vi "Background_MC_Acquire_v2.vi"(7 "prev deleted portion":u16[](array[numeric]), 8 "error in":errorcluster, 9 "Image In":T2, 10 "Frames":i16, 11 "FPGA VI Reference In":T1) -> (0 "error out":errorcluster, 1 "deleted portion":u16[](array[numeric]), 2 "Image":T2(plugin-control), 3 "FPGA VI Reference Out":T1)   [LabVIEW 2020]
uses:
  RIG-SPECIFIC FILES/FPGA Refs/FPGA Ref.ctl
  <vilib>/vision/Image Controls.llb/IMAQ Image.ctl
  <vilib>/Utility/error.llb/Error Cluster From Error Code.vi
  <vilib>/rvi/errors/niLvFpgaAdjustHostInterfaceError.vi
  <vilib>/rvi/interface/nirviMethod/nirviMethod.xnode
  <vilib>/FPGAPlugInAG/Dynamic/niLvFpga_ReadFifo_Dynamic.vi
  <vilib>/rvi/errors/niLvFpgaMergeErrorWithErrorCode.vi
panel:
  out "deleted ele":i32
  out "1D Array incoming":i32
  out "1D Array size Adj":i32(graph)
  out "1D Array incoming":cluster{"Total number of pixels":i16, i32}(graph)
  out "Final Array size":i32[](array[numeric])
  out "Reshaped Array size":i32[](array[numeric])
  out "1D Array size":i32
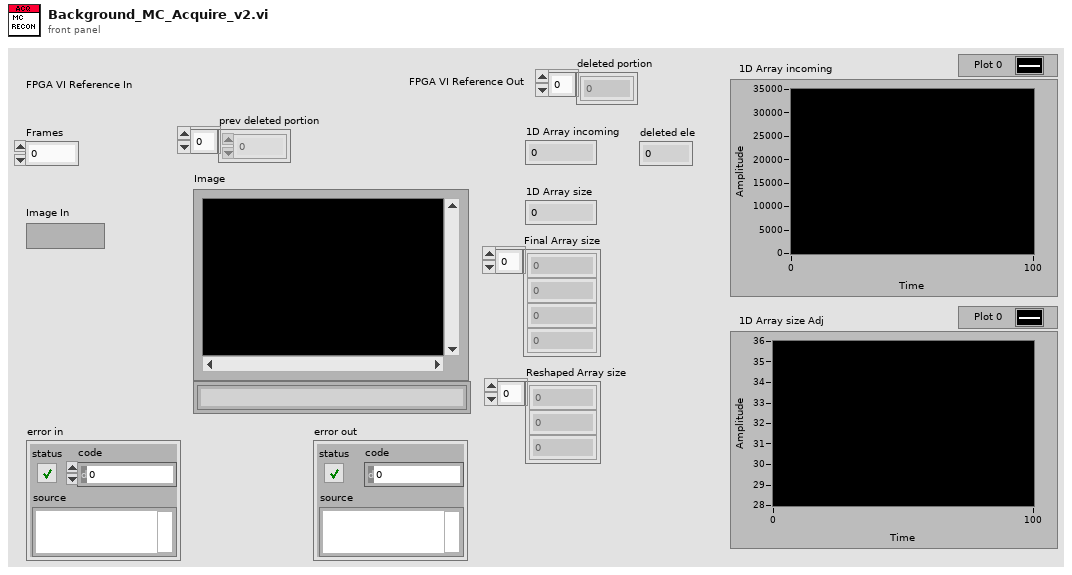
[diagram p1: front panel]
types:
  T1 = typedef "FPGA Ref.ctl" = refnum<k20>
  T2 = typedef "IMAQ Image.ctl" = refnum<image>
  T3 = typedef "Ref DAQ Param.ctl" = cluster{"Full Frame Size":u16, "Ref Field of View":sgl, "Ref Zoom":i8, "Ref_dwellTime":sgl, "Ref X-pixels-per-line(Npxr)":i16, "Ref Y-lines-per-image(Npyr)":i16, "Ref Z-lines-per-image":i16, "Ignore Z lines":i16, "Ref Scan Cycles":i32, "Ref threshold XY":u16, "Ref threshold Z":u16, "Ref average XY":u16, "Ref Average  Z":u16, "Proportional_scale":fxp<+,16,2>, "Integral_scale":fxp<+/-,16,12>, "Proportional_scale Z":fxp<+,16,2>, "Integral_scale Z":fxp<+/-,16,12>, "Diff_threshold":fxp<+,16,2>, "Diff_threshold _z":fxp<+,16,2>, "Sliding Average":bool, "Ref count reset enabled":bool, "Auto-centering":bool}
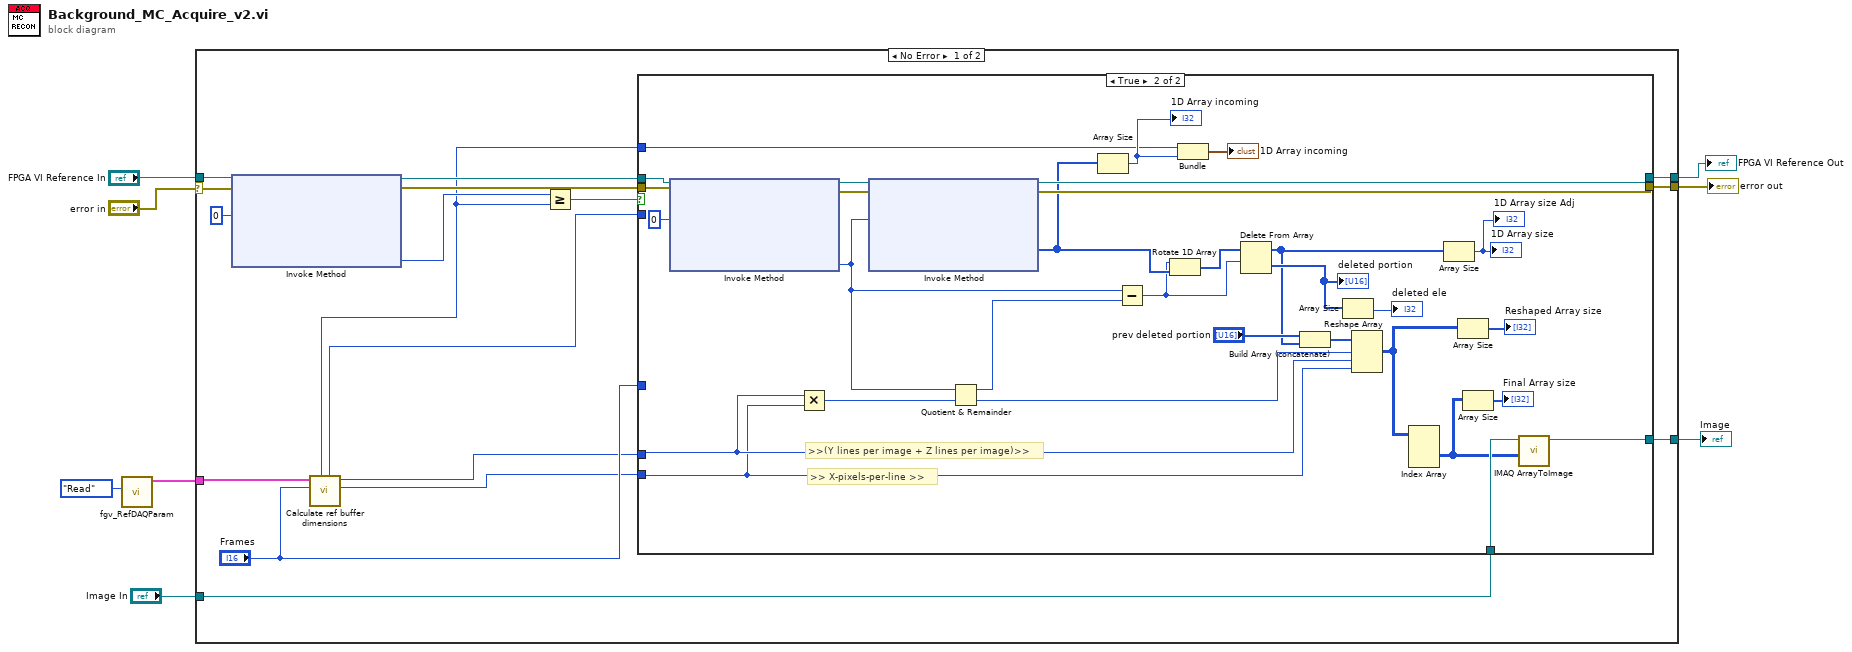
[diagram p0: block diagram]
diagram:
  n1 = call "fgv_RefDAQParam.vi"("Function"=enum16{"Initialize", "Write", "Read"}."Read") -> ("RefDAQParam"=w5:T3)  [unwired: 9 in, 1 out]
  n2 = case shown="No Error" "error in" {
    selector: "error in" -> [w23 w59]
    tunnel: "FPGA VI Reference In" -> [w25 w60]
    tunnel: w5 -> [w18 _]
    tunnel: "Image In" -> [w13 w61]
    tunnel: [w12 w61] -> w3
    tunnel: [w11 w60] -> w2
    tunnel: [w10 w59] -> w1
    frame No Error {
      n3 = xnode "Invoke Method"("FPGA VI Reference In"=w25, "error in"=w23, "Number of Elements"=u32 0) -> ("FPGA VI Reference Out"=w20:T1, "error out"=w19:errorcluster, "Elements Remaining"=w22:u32)  [unwired: 1 in, 1 out]
      n4 = call "Calculate ref buffer dimensions.vi"("Frames"="Frames", "RefDAQParam in"=w18) -> ("Ref X-pixels-per-line(Npxr)"=w14:i16, "Y lines  + Z lines"=w15:i16, "Number of pixels per frame"=w16:i16, "Total number of pixels"=w9:i16)  [unwired: 4 in, 2 out]
      n5 = Greater Or Equal?(x=w22, y=w9) -> (x >= y?=w21:bool)
      n6 = case shown="True" w21 {
        tunnel: w20 -> [w28 w52]
        tunnel: w19 -> [w27 w58]
        tunnel: w16 -> [_ _]
        tunnel: "Frames" -> [_ _]
        tunnel: w15 -> [_ w47]
        tunnel: w14 -> [_ w46]
        tunnel: w13 -> [w26 w57]
        tunnel: [w26 w56] -> w12
        tunnel: [w28 w55] -> w11
        tunnel: [w27 w54] -> w10
        tunnel: w9 -> [_ w42]
        frame False {
        }
        frame True {
          # ">>(Y lines per image + Z lines per image)>>"
          # ">> X-pixels-per-line >>"
          n7 = xnode "Invoke Method"("FPGA VI Reference In"=w52, "Number of Elements"=u32 0) -> ("FPGA VI Reference Out"=w53:T1, "Elements Remaining"=w34:u32)  [unwired: 2 in, 2 out]
          n8 = Multiply(x=w47, y=w46) -> (x*y=w35:i16)
          n9 = xnode "Invoke Method"("FPGA VI Reference In"=w53, "error in"=w58, "Number of Elements"=w34) -> ("FPGA VI Reference Out"=w55:T1, "error out"=w54:errorcluster, "Data"=w38:u16[])  [unwired: 1 in, 1 out]
          n10 = Quotient & Remainder(x=w34, y=w35) -> (x-y*floor(x/y)=w33:u32, floor(x/y)=w32:u32)
          n11 = Array Size(array=w38) -> (size(s)=w43:i32)
          "1D Array incoming" <- w43
          n12 = Subtract(x=w34, y=w33) -> (x-y=w36:u32)
          n13 = Rotate 1D Array(1:w38, 2:w36) -> (0:w37:u16[])
          n14 = Bundle("Total number of pixels"=w42, w43) -> (→"1D Array incoming":cluster{"Total number of pixels":i16, i32})  [unwired: 1 in]
          n15 = Delete From Array(array=w37, length=w36) -> (deleted portion=w40:u16[], array with subset deleted=w29:u16[])  [unwired: 1 in]
          "deleted portion" <- w40
          n16 = Build Array (concatenate)("prev deleted portion", w29) -> (w31:u16[])
          n17 = Array Size(array=w40) -> (size(s)=→"deleted ele":i32)
          n18 = Reshape Array(w31, w32, w47, w46) -> (w50:u16[][][])
          n19 = Index Array(array=w50) -> (element=w45:u16[][])  [unwired: 3 in]
          n20 = Array Size(array=w29) -> (size(s)=→"1D Array size" →"1D Array size Adj":i32)
          n21 = Array Size(array=w50) -> (size(s)=→"Reshaped Array size":i32[])
          n22 = Array Size(array=w45) -> (size(s)=→"Final Array size":i32[])
          n23 = call "IMAQ ArrayToImage"("Image Pixels (I16)"=w45, "Image"=w57) -> ("Image Out"=w56:T2)  [unwired: 8 in, 1 out]
        }
      }
    }
    frame Error {
    }
  }
  "Image" <- w3
  "FPGA VI Reference Out" <- w2
  "error out" <- w1
